vi "AG34980A_Configure_DC_Voltage.vi"(0 "VISA resource name":refnum<visa-resource-name>, 2 "Input Impedance (F:Fixed)":bool, 5 "Range (5:Auto)":T1(ring)=enum."Auto", 7 "Resolution (5:Default)":T2(ring)=enum."Default", 9 "Autozero (0:ON)":enum16{"On", "Off", "Once"}(ring), 11 "error in (no error)":errorcluster) -> (4 "VISA resource name out":refnum<visa-resource-name>, 15 "error out":errorcluster)   [LabVIEW 2022 SP3, in "DMM_Keysight_34980A.lvlib" / "DMM_Keysight_34980A.lvclass"]
doc: "This VI allows you to control various settings for performing DC voltage measurements. You can independently specify the range, resolution, autozero mode, and input impedance."
uses:
  DMM_Keysight_34980A.lvclass
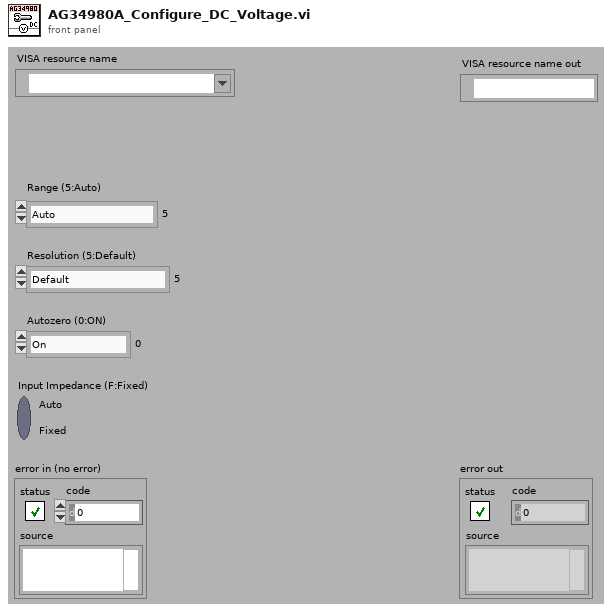
[diagram p1: front panel]
types:
  T1 = enum16{"100 mV", "1 V", "10 V", "100 V", "300 V", "Auto", "Minimum", "Maximum"}
  T2 = enum16{"4 1/2", "5 1/2", "6 1/2", "Least", "Highest", "Default"}
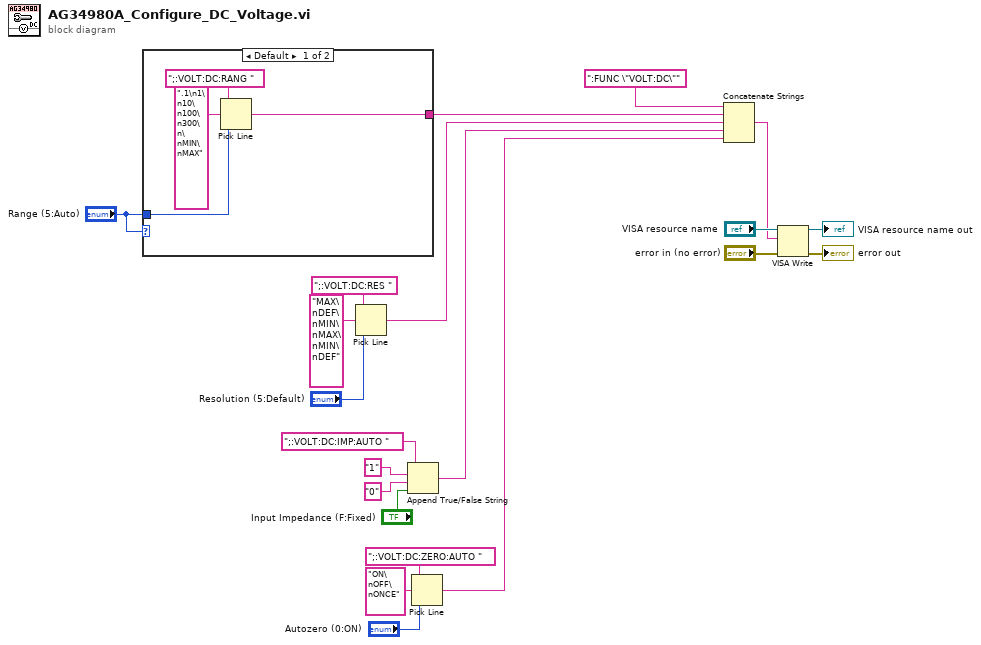
[diagram p0: block diagram]
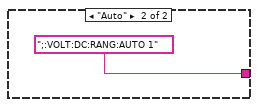
[diagram p2: hidden frame]
diagram:
  n1 = case shown="Default" "Range (5:Auto)" {
    tunnel: "Range (5:Auto)" -> [w23 _]
    tunnel: [w22 ";:VOLT:DC:RANG:AUTO 1"] -> w21
    frame Default {
      n2 = Pick Line(string ("")=";:VOLT:DC:RANG ", multi-line string=".1\n1\n10\n100\n300\n\nMIN\nMAX", line index=w23) -> (output string=w22:string)
    }
    frame "Auto" {
    }
  }
  n3 = Pick Line(string ("")=";:VOLT:DC:RES ", multi-line string="MAX\nDEF\nMIN\nMAX\nMIN\nDEF", line index="Resolution (5:Default)") -> (output string=w1:string)
  n4 = Append True/False String(1:"Input Impedance (F:Fixed)", 2:"0", 3:"1", 4:";:VOLT:DC:IMP:AUTO ") -> (0:w10:string)
  n5 = Pick Line(string ("")=";:VOLT:DC:ZERO:AUTO ", multi-line string="ON\nOFF\nONCE", line index="Autozero (0:ON)") -> (output string=w6:string)
  n6 = Concatenate Strings(":FUNC \"VOLT:DC\"", w21, w1, w10, w6) -> (w16:string)
  n7 = VISA Write(VISA resource name="VISA resource name", write buffer=w16, error in (no error)="error in (no error)") -> (VISA resource name out=→"VISA resource name out":refnum<visa-resource-name>, error out=→"error out":errorcluster)  [unwired: 1 out]
